vi "Convex Hull 2D (GiftWrap) with area and perimeter output.vi"(0 "STL file path":path=path "C:/EnFlo_Data_Local/Preferences/Rig_Setups/EnFlo_Tunnel/All_Users/Collision_detection/Model/MAGIC_London_Southbank_0_deg_excl_12_and_150.stl", 1 "Flatten to plane":u8(ring) items=["XY", "XZ", "YZ"], 2 "epsilon (model units)":sgl=0.001) -> (3 "Convex hull lines":T1[](array[typedef])=[{"V0"=[2107.238, -278.4084, 0.0], "V1"=[2160.1506, 148.22986, 0.0], "i0"=378, "i1"=348}, {"V0"=[2160.1506, 148.22986, 0.0], "V1"=[2143.7957, 256.90976, 0.0], "i0"=348, "i1"=341}, {"V0"=[2143.7957, 256.90976, 0.0], "V1"=[1743.7455, 1101.0426, 0.0], "i0"=341, "i1"=338}, {"V0"=[1743.7455, 1101.0426, 0.0], "V1"=[1683.7944, 1209.5332, 0.0], "i0"=338, "i1"=337}, {"V0"=[1683.7944, 1209.5332, 0.0], "V1"=[-498.39395, 2003.7932, 0.0], "i0"=337, "i1"=27}, {"V0"=[-498.39395, 2003.7932, 0.0], "V1"=[-695.90735, 1993.0829, 0.0], "i0"=27, "i1"=28}, {"V0"=[-695.90735, 1993.0829, 0.0], "V1"=[-920.447, 1921.0448, 0.0], "i0"=28, "i1"=25}, {"V0"=[-920.447, 1921.0448, 0.0], "V1"=[-1520.1244, 807.2517, 0.0], "i0"=25, "i1"=272}, {"V0"=[-1520.1244, 807.2517, 0.0], "V1"=[-1574.2631, 642.39484, 0.0], "i0"=272, "i1"=277}, {"V0"=[-1574.2631, 642.39484, 0.0], "V1"=[-1612.0717, 236.09502, 0.0], "i0"=277, "i1"=72}, {"V0"=[-1612.0717, 236.09502, 0.0], "V1"=[-1334.8026, -1485.3105, 0.0], "i0"=72, "i1"=721}, {"V0"=[-1334.8026, -1485.3105, 0.0], "V1"=[-1225.0652, -1688.8436, 0.0], "i0"=721, "i1"=719}, {"V0"=[-1225.0652, -1688.8436, 0.0], "V1"=[-406.50937, -2046.7448, 0.0], "i0"=719, "i1"=581}, {"V0"=[-406.50937, -2046.7448, 0.0], "V1"=[563.3067, -2329.1704, 0.0], "i0"=581, "i1"=230}, {"V0"=[563.3067, -2329.1704, 0.0], "V1"=[743.1804, -2109.3914, 0.0], "i0"=230, "i1"=231}, {"V0"=[743.1804, -2109.3914, 0.0], "V1"=[1808.6718, -718.93787, 0.0], "i0"=231, "i1"=544}, {"V0"=[1808.6718, -718.93787, 0.0], "V1"=[2055.1643, -355.62637, 0.0], "i0"=544, "i1"=379}, {"V0"=[2055.1643, -355.62637, 0.0], "V1"=[2107.238, -278.4084, 0.0], "i0"=379, "i1"=378}], 4 "Convex hull vertices":sgl[][](array[numeric])=[[2160.1506, 148.22986, 0.0], [2143.7957, 256.90976, 0.0], [1743.7455, 1101.0426, 0.0], [1683.7944, 1209.5332, 0.0], [-498.39395, 2003.7932, 0.0], [-695.90735, 1993.0829, 0.0], [-920.447, 1921.0448, 0.0], [-1520.1244, 807.2517, 0.0], [-1574.2631, 642.39484, 0.0], [-1612.0717, 236.09502, 0.0], [-1334.8026, -1485.3105, 0.0], [-1225.0652, -1688.8436, 0.0], [-406.50937, -2046.7448, 0.0], [563.3067, -2329.1704, 0.0], [743.1804, -2109.3914, 0.0], [1808.6718, -718.93787, 0.0], [2055.1643, -355.62637, 0.0], [2107.238, -278.4084, 0.0]], 5 "Convex hull perimeter (model units)":sgl=12646.526, 6 "Convex hull area (model units^2)":sgl=11614809.0)   [LabVIEW 2016]
uses:
  Typedefs/Edge, indexed.ctl
  Subroutines/Coincident points test.vi
panel:
  out "Convex hull vertices (model units)":string="X\tY\tZ\r\n2160.1506\t148.2299\t0.0000\r\n2143.7957\t256.9098\t0.0000\r\n1743.7455\t1101.0426\t0.0000\r\n1683.7944\t1209.5332\t0.0000\r\n-498.3940\t2003.7932\t0.0000\r\n-695.9073\t1993.0829\t0.0000\r\n-920.4470\t1921.0448\t0.0000\r\n-1520.1244\t807.2517\t0.0000\r\n-1574.2631\t642.3948\t0.0000\r\n-1612.0717\t236.0950\t0.0000\r\n-1334.8026\t-1485.3105\t0.0000\r\n-1225.0652\t-1688.8436\t0.0000\r\n-406.5094\t-2046.7448\t0.0000\r\n563.3067\t-2329.1704\t0.0000\r\n743.1804\t-2109.3914\t0.0000\r\n1808.6718\t-718.9379\t0.0000\r\n2055.1643\t-355.6264\t0.0000\r\n2107.2380\t-278.4084\t0.0000\r\n"
  out "Visualisation":cluster{sgl[], sgl[]}[](graph)=[{array[722 elements], array[722 elements]}, {[2107.238, 2160.1506], [-278.4084, 148.22986]}, {[2160.1506, 2143.7957], [148.22986, 256.90976]}, {[2143.7957, 1743.7455], [256.90976, 1101.0426]}, {[1743.7455, 1683.7944], [1101.0426, 1209.5332]}, {[1683.7944, -498.39395], [1209.5332, 2003.7932]}, {[-498.39395, -695.90735], [2003.7932, 1993.0829]}, {[-695.90735, -920.447], [1993.0829, 1921.0448]}, {[-920.447, -1520.1244], [1921.0448, 807.2517]}, {[-1520.1244, -1574.2631], [807.2517, 642.39484]}, {[-1574.2631, -1612.0717], [642.39484, 236.09502]}, {[-1612.0717, -1334.8026], [236.09502, -1485.3105]}, {[-1334.8026, -1225.0652], [-1485.3105, -1688.8436]}, {[-1225.0652, -406.50937], [-1688.8436, -2046.7448]}, {[-406.50937, 563.3067], [-2046.7448, -2329.1704]}, {[563.3067, 743.1804], [-2329.1704, -2109.3914]}, {[743.1804, 1808.6718], [-2109.3914, -718.93787]}, {[1808.6718, 2055.1643], [-718.93787, -355.62637]}, {[2055.1643, 2107.238], [-355.62637, -278.4084]}]
  # "PN 11/08/2017"
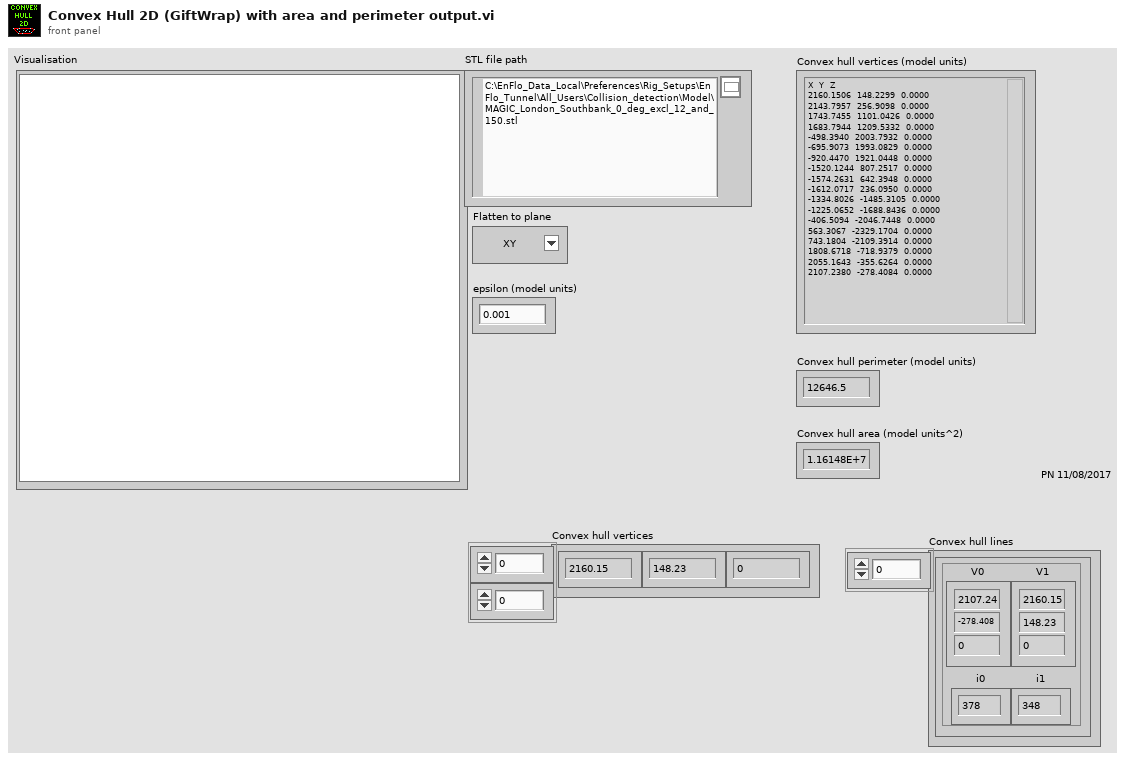
[diagram p1: front panel]
types:
  T1 = typedef "Edge, indexed.ctl" = cluster{"V0":sgl[], "V1":sgl[], "i0":i32, "i1":i32}
  T2 = typedef "Triangle.ctl" = cluster{"V0":sgl[], "V1":sgl[], "V2":sgl[], "E0":sgl[], "E1":sgl[], "E2":sgl[], "n^":sgl[], "nE0^":sgl[], "nE1^":sgl[], "nE2^":sgl[]}
  T3 = cluster{"Vertices (without duplicates)":sgl[], "Vertices (without duplicates)":sgl[]}
  T4 = cluster{"Vertices (without duplicates)":sgl[], "Vertices (without duplicates)":sgl[]}[]
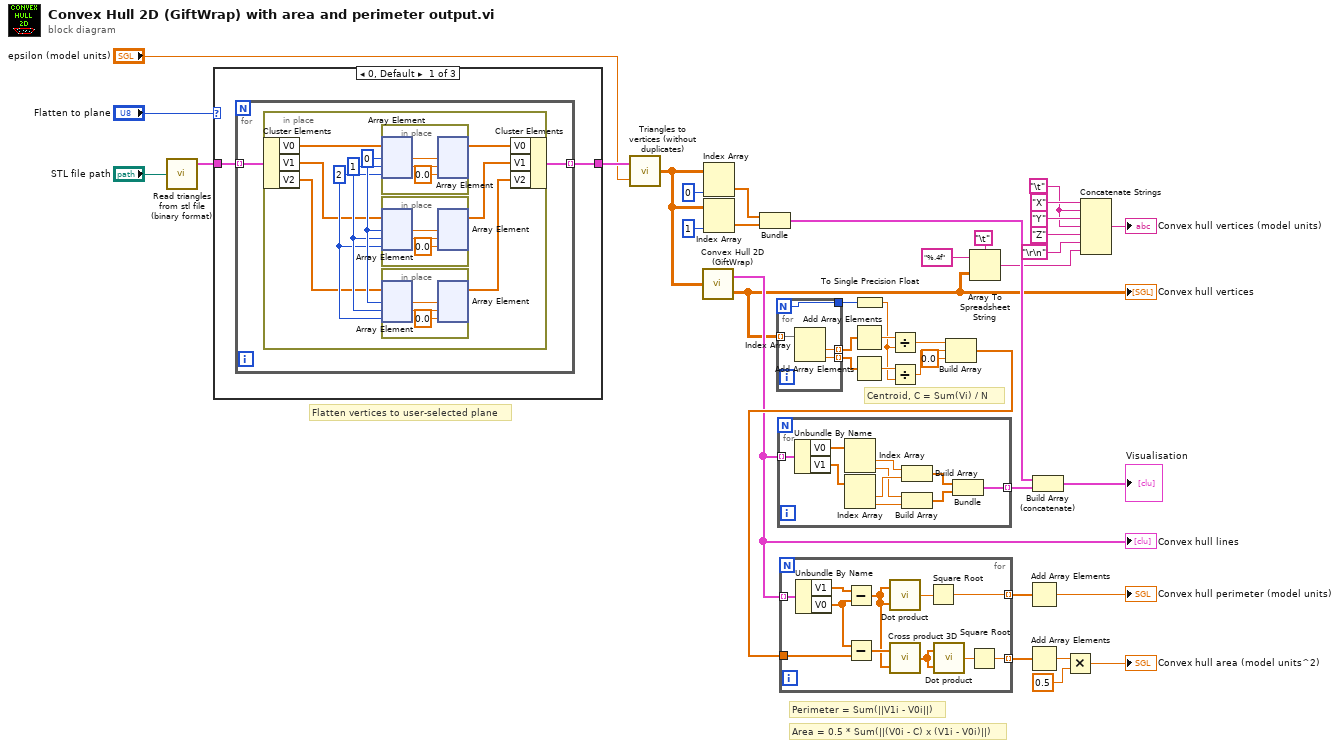
[diagram p0: block diagram]
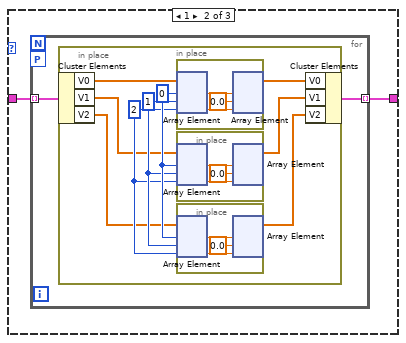
[diagram p2: hidden frame]
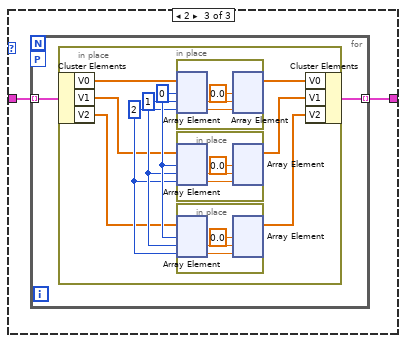
[diagram p3: hidden frame]
diagram:
  w23 = "\t"
  # "Perimeter = Sum(||V1i - V0i||)"
  # "Area = 0.5 * Sum(||(V0i - C) x (V1i - V0i)||)"
  # "Centroid, C = Sum(Vi) / N"
  # "Flatten vertices to user-selected plane"
  n1 = call "Read triangles from stl file (binary format).vi"("STL file path"="STL file path") -> ("Triangles array"=w20:T2[])  [unwired: 2 out]
  n2 = case shown="0, Default" "Flatten to plane" {
    tunnel: [w42 w64 w86] -> w19
    tunnel: w20 -> [w41 w63 w85]
    frame 0, Default {
      n3 = for {
        tunnel: w41 -> [w44] mode=indexing
        tunnel: [w43] -> w42 mode=indexing
        n4 = in-place {
          w51 = 2
          w52 = 1
          w53 = 0
          n5 = in-place-cluster #1(w44) -> ("V0"=w50:sgl[], "V1"=w49:sgl[], "V2"=w48:sgl[])
          n6 = in-place {
            n7 = in-place-array #2(w50, w53, w52, w51) -> (w62:sgl, w61:sgl)  [unwired: 1 out]
            n8 = in-place-array #2(w62, w61, sgl 0.0 ("element")) -> (w47:sgl[])  [unwired: 3 out]
          }
          n9 = in-place {
            n10 = in-place-array #3(w49, w53, w52, w51) -> (w59:sgl, w58:sgl)  [unwired: 1 out]
            n11 = in-place-array #3(w59, w58, sgl 0.0 ("element")) -> (w46:sgl[])  [unwired: 3 out]
          }
          n12 = in-place {
            n13 = in-place-array #4(w48, w53, w52, w51) -> (w56:sgl, w55:sgl)  [unwired: 1 out]
            n14 = in-place-array #4(w56, w55, sgl 0.0 ("element")) -> (w45:sgl[])  [unwired: 3 out]
          }
          n15 = in-place-cluster #1("V0"=w47, "V1"=w46, "V2"=w45) -> (w43:T2)
        }
      }
    }
    frame 1 {
      n16 = for {
        tunnel: w63 -> [w66] mode=indexing
        tunnel: [w65] -> w64 mode=indexing
        workers-P: _ -> [_]
        n17 = in-place {
          w73 = 2
          w74 = 1
          w75 = 0
          n18 = in-place-cluster #5(w66) -> ("V0"=w72:sgl[], "V1"=w71:sgl[], "V2"=w70:sgl[])
          n19 = in-place {
            n20 = in-place-array #6(w72, w75, w74, w73) -> (w84:sgl, w82:sgl)  [unwired: 1 out]
            n21 = in-place-array #6(w84, sgl 0.0 ("element"), w82) -> (w69:sgl[])  [unwired: 3 out]
          }
          n22 = in-place {
            n23 = in-place-array #7(w71, w75, w74, w73) -> (w81:sgl, w79:sgl)  [unwired: 1 out]
            n24 = in-place-array #7(w81, sgl 0.0 ("element"), w79) -> (w68:sgl[])  [unwired: 3 out]
          }
          n25 = in-place {
            n26 = in-place-array #8(w70, w75, w74, w73) -> (w78:sgl, w76:sgl)  [unwired: 1 out]
            n27 = in-place-array #8(w78, sgl 0.0 ("element"), w76) -> (w67:sgl[])  [unwired: 3 out]
          }
          n28 = in-place-cluster #5("V0"=w69, "V1"=w68, "V2"=w67) -> (w65:T2)
        }
      }
    }
    frame 2 {
      n29 = for {
        tunnel: w85 -> [w88] mode=indexing
        tunnel: [w87] -> w86 mode=indexing
        workers-P: _ -> [_]
        n30 = in-place {
          w95 = 2
          w96 = 1
          w97 = 0
          n31 = in-place-cluster #9(w88) -> ("V0"=w94:sgl[], "V1"=w93:sgl[], "V2"=w92:sgl[])
          n32 = in-place {
            n33 = in-place-array #10(w94, w97, w96, w95) -> (w106:sgl, w104:sgl)  [unwired: 1 out]
            n34 = in-place-array #10(sgl 0.0 ("element"), w106, w104) -> (w91:sgl[])  [unwired: 3 out]
          }
          n35 = in-place {
            n36 = in-place-array #11(w93, w97, w96, w95) -> (w103:sgl, w101:sgl)  [unwired: 1 out]
            n37 = in-place-array #11(sgl 0.0 ("element"), w103, w101) -> (w90:sgl[])  [unwired: 3 out]
          }
          n38 = in-place {
            n39 = in-place-array #12(w92, w97, w96, w95) -> (w100:sgl, w98:sgl)  [unwired: 1 out]
            n40 = in-place-array #12(sgl 0.0 ("element"), w100, w98) -> (w89:sgl[])  [unwired: 3 out]
          }
          n41 = in-place-cluster #9("V0"=w91, "V1"=w90, "V2"=w89) -> (w87:T2)
        }
      }
    }
  }
  n42 = call "Triangles to vertices (without duplicates).vi"("epsilon"="epsilon (model units)", "Triangles"=w19) -> ("Vertices (without duplicates)"=w3:sgl[][])
  n43 = call "Convex Hull 2D (GiftWrap).vi"("Points"=w3) -> ("Convex Hull lines"=w2:T1[], "Convex Hull vertices"=w1:sgl[][])
  "Convex hull vertices" <- w1
  "Convex hull lines" <- w2
  n44 = Index Array(array=w3, index (col)=0 ("disabled index (col)")) -> (element=w36:sgl[])  [unwired: 1 in]
  n45 = Index Array(array=w3, index (col)=1 ("disabled index (col)")) -> (element=w34:sgl[])  [unwired: 1 in]
  n46 = Bundle("Vertices (without duplicates)"=w36, "Vertices (without duplicates)"=w34) -> (w38:T3)  [unwired: 1 in]
  n47 = for {
    N -> [w107]
    tunnel: w1 -> [w110] mode=indexing
    tunnel: [w109] -> w18 mode=indexing
    tunnel: [w108] -> w17 mode=indexing
    tunnel: [w107] -> w14
    n48 = Index Array(array=w110) -> (element #1=w109:sgl, element #2=w108:sgl)  [unwired: 2 in]
  }
  n49 = for {
    tunnel: [w112] -> w39 mode=indexing
    tunnel: w2 -> [w111] mode=indexing
    n50 = Unbundle By Name(w111) -> ("V0"=w114:sgl[], "V1"=w113:sgl[])
    n51 = Index Array(array=w114) -> (element #1=w120:sgl, element #2=w117:sgl)  [unwired: 2 in]
    n52 = Index Array(array=w113) -> (element #1=w118:sgl, element #2=w116:sgl)  [unwired: 2 in]
    n53 = Build Array(w120, w118) -> (w119:sgl[])
    n54 = Build Array(w117, w116) -> (w115:sgl[])
    n55 = Bundle(w119, w115) -> (w112:cluster{sgl[], sgl[]})  [unwired: 1 in]
  }
  n56 = Add Array Elements(numeric array=w18) -> (sum=w15:sgl)
  n57 = Add Array Elements(numeric array=w17) -> (sum=w16:sgl)
  n58 = To Single Precision Float(number=w14) -> (single precision float=w13:sgl)
  n59 = Divide(x=w15, y=w13) -> (x/y=w11:sgl)
  n60 = Divide(x=w16, y=w13) -> (x/y=w10:sgl)
  n61 = Build Array(w11, w10, sgl 0.0 ("element")) -> (w9:sgl[])
  n62 = for {
    tunnel: w2 -> [w131] mode=indexing
    tunnel: [w129] -> w22 mode=indexing
    tunnel: w9 -> [w127]
    tunnel: [w121] -> w8 mode=indexing
    n63 = Unbundle By Name(w131) -> ("V1"=w126:sgl[], "V0"=w128:sgl[])
    n64 = Subtract(x=w126, y=w128) -> (x-y=w124:sgl[])
    n65 = Subtract(x=w128, y=w127) -> (x-y=w125:sgl[])
    n66 = call "Dot product.vi"("B"=w124, "A"=w124) -> ("A . B"=w130:sgl)
    n67 = call "Cross product 3D.vi"("B"=w124, "A"=w125) -> ("A x B"=w123:sgl[])
    n68 = Square Root(x=w130) -> (sqrt(x)=w129:sgl)
    n69 = call "Dot product.vi"("B"=w123, "A"=w123) -> ("A . B"=w122:sgl)
    n70 = Square Root(x=w122) -> (sqrt(x)=w121:sgl)
  }
  n71 = Array To Spreadsheet String(delimiter (Tab)="\t", array=w1, 3:"%.4f" ("format string")) -> (spreadsheet string=w24:string)
  n72 = Add Array Elements(numeric array=w22) -> (sum=→"Convex hull perimeter (model units)":sgl)
  n73 = Add Array Elements(numeric array=w8) -> (sum=w7:sgl)
  n74 = Build Array (concatenate)(w38, w39) -> (→"Visualisation":T4)
  n75 = Multiply(x=w7, y=sgl 0.5) -> (x*y=→"Convex hull area (model units^2)":sgl)
  n76 = Concatenate Strings("X", w23, "Y", w23, "Z", "\r\n", w24) -> (→"Convex hull vertices (model units)":string)
